vi "DHE_ResetexposureID.vi"(8 "error in (no error)":errorcluster) -> (0 "error out":errorcluster)   [LabVIEW 2016]
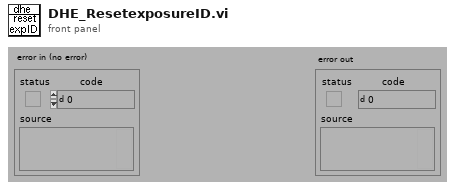
[diagram p1: front panel]
types:
  T1 = typedef "DatabaseHand_RefNum.ctl" = refnum<vi>
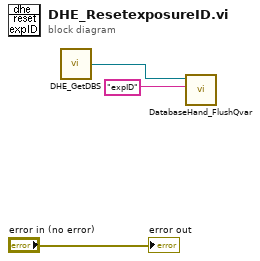
[diagram p0: block diagram]
diagram:
  n1 = call "DHE_GetDBS.vi"() -> ("DHE_DBSRef"=w1:T1)  [unwired: 9 out]
  n2 = call "DatabaseHand_FlushQvar.vi"("name"="expID", "Database RefNum In"=w1) -> ()  [unwired: 1 in, 9 out]
  "error out" <- "error in (no error)"
